vi "Read Last error.vi"(8 "error in (no error)":errorcluster, 11 "RP Communicator in":refnum<class "RP Communicator.lvclass">) -> (0 "error out":errorcluster, 2 "Last error":errorcluster, 3 "RP Communicator out":refnum<class "RP Communicator.lvclass">)   [LabVIEW 2021, in "RP Communicator.lvclass"]
uses:
  RP Communicator.lvclass
  RP Communicator.lvclass/RP Communicator.ctl
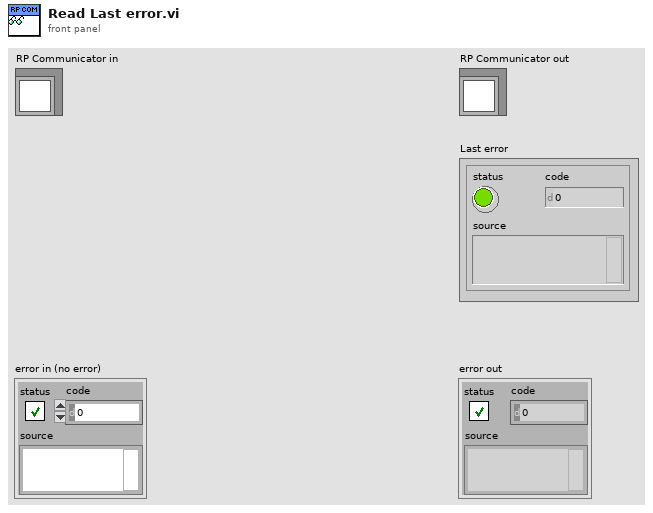
[diagram p1: front panel]
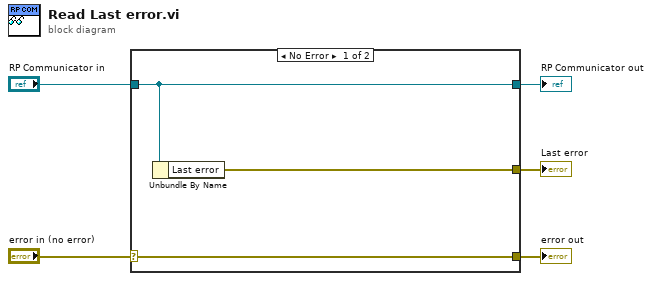
[diagram p0: block diagram]
diagram:
  n1 = case shown="No Error" "error in (no error)" {
    selector: "error in (no error)" -> [w8 w9]
    tunnel: [w8 w9] -> w4
    tunnel: [w7 w10] -> w2
    tunnel: "RP Communicator in" -> [w7 w10]
    tunnel: [w6 _] -> w1
    frame No Error {
      n2 = Unbundle By Name(w7) -> ("Last error"=w6:errorcluster)
    }
    frame Error {
    }
  }
  "error out" <- w4
  "RP Communicator out" <- w2
  "Last error" <- w1
